vi "Analog Output Data Generation.vi"(3 "AO Timing":T1={"samples per channel"=1000, "sample mode"=10178, "Sampling Rate"=1000.0} {"sample mode" items=["Finite Samples"=10178, "Continuous Samples"=10123, "Hardware Timed Single Point"=12522]}, 4 "Configuration Data":T2[](array[typedef]), 5 "6738 Card?":bool, 6 "Path":path, 7 "AO Task":refnum<k21>, 8 "error in":errorcluster, 9 "Stop Notifier":refnum<notifier>, 10 "Main Engine Respons  Q":refnum<queue>, 11 "Interupt Q":refnum<queue>) -> (0 "error out":errorcluster, 2 "All Stop":bool)   [LabVIEW 2024]
doc: "All Rights Reserved © 2017 SyncSols"
uses:
  TCP Engine/Controls/TCP Engine I&O  Interupt Cluster.ctl
  Controls/AO Channel Configuration Cluster.ctl
  Controls/AO Timing Cluster.ctl
  <vilib>/DAQmx/write.llb/DAQmx Write (Analog 1D Wfm NChan NSamp).vi
  <vilib>/DAQmx/miscellaneous.llb/DAQmx Fill In Error Info.vi
  TCP Engine/TCP Engine.lvlib
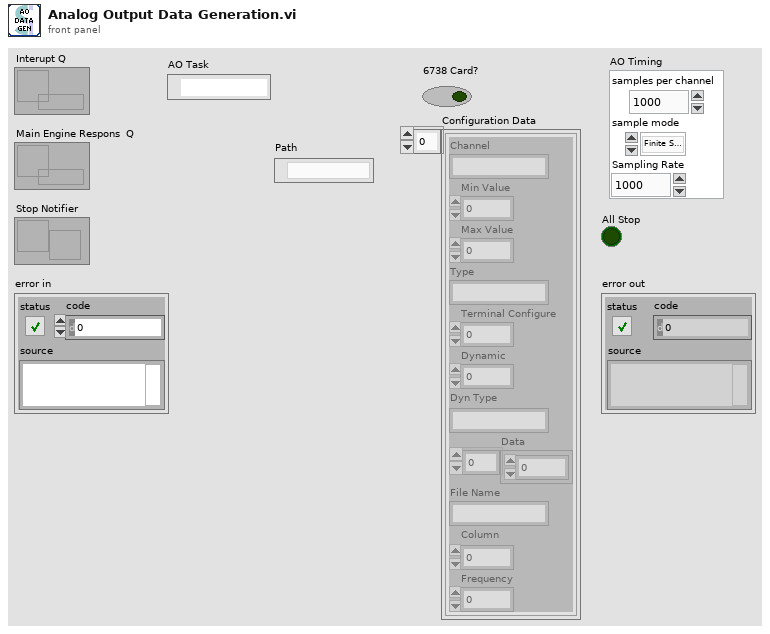
[diagram p1: front panel]
types:
  T1 = typedef "AO Timing Cluster.ctl" = cluster{"samples per channel":i32, "sample mode":i32, "Sampling Rate":dbl}
  T2 = typedef "AO Channel Configuration Cluster.ctl" = cluster{"Channel":string, "Min Value":dbl, "Max Value":dbl, "Type":string, "Terminal Configure":u16, "Dynamic":u8, "Dyn Type":string, "Data":dbl[], "File Name":string, "Column":i32, "Frequency":dbl}
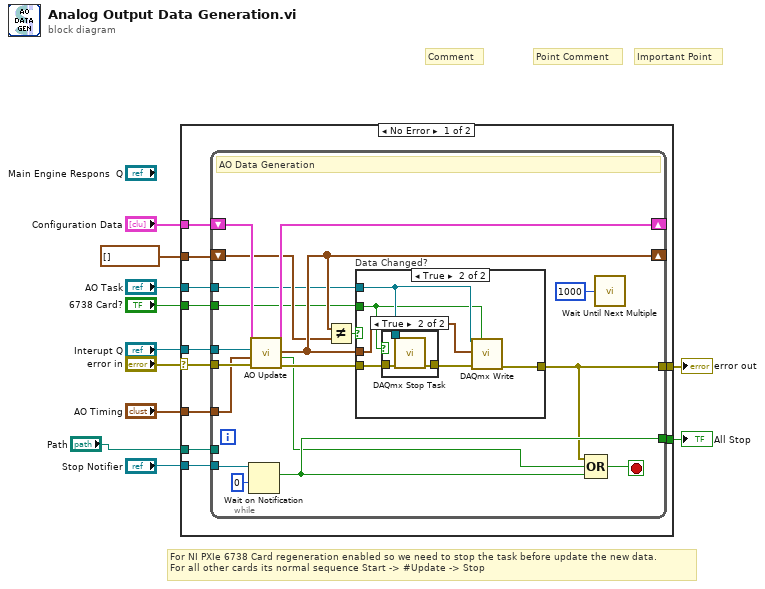
[diagram p0: block diagram]
diagram:
  # "For NI PXIe 6738 Card regeneration enabled so we need to stop the task before update the new data.\nFor all other cards its normal sequence Start -> #Update -> Stop"
  # "Important Point"
  # "Point Comment"
  # "Comment"
  n1 = case shown="No Error" "error in" {
    selector: "error in" -> [w20 w52]
    tunnel: [w18 w52] -> w11
    tunnel: "Stop Notifier" -> [w22 _]
    tunnel: "Interupt Q" -> [w21 _]
    tunnel: "AO Task" -> [w19 _]
    tunnel: "Path" -> [w17 _]
    tunnel: [w16 _] -> w7
    tunnel: "Configuration Data" -> [w15 _]
    tunnel: "AO Timing" -> [w14 _]
    tunnel: waveform(dbl)[] [] ("Data To Generate") -> [w13 _]
    tunnel: "6738 Card?" -> [w12 _]
    frame No Error {
      n2 = while {
        tunnel: w22 -> [w40]
        tunnel: w21 -> [w33]
        tunnel: w20 -> [w35]
        tunnel: w19 -> [w24]
        tunnel: [w29] -> w18
        tunnel: w17 -> [_]
        tunnel: [w37] -> w16
        tunnel: w14 -> [w32]
        shift-right: [w30] -> _
        shift-left: w15 -> [w34]
        shift-right: [w27] -> _
        shift-left: w13 -> [w26]
        tunnel: w12 -> [w23]
        stop <- w38 stop-if-true
        # "AO Data Generation"
        n3 = Wait on Notification(notifier=w40, timeout in ms (-1)=0) -> (notification=w37:bool)  [unwired: 2 in, 3 out]
        n4 = call "AO Update.vi"("error in"=w35, "AO Timing"=w32, "Interupt Q"=w33, "Configuration Data"=w34) -> ("error out"=w36:errorcluster, "Stop"=w31:bool, "Data To Generate"=w27:waveform(dbl)[], "Configuration Data"=w30:T2[])  [unwired: 4 in]
        n5 = Not Equal?(x=w27, y=w26) -> (x != y?=w28:bool)
        n6 = case "Data Changed?" shown="True" w28 {
          tunnel: w24 -> [_ w44]
          tunnel: w36 -> [w41 w45]
          tunnel: [w41 w47] -> w29
          tunnel: w27 -> [_ w46]
          tunnel: w23 -> [_ w42]
          frame False {
          }
          frame True {
            n7 = case shown="True" w42 {
              tunnel: w45 -> [w48 w51]
              tunnel: w44 -> [_ w50]
              tunnel: [w48 w49] -> w43
              frame False {
              }
              frame True {
                n8 = call <vilib>:"DAQmx Stop Task.vi"("task/channels in"=w50, "error in"=w51) -> ("error out"=w49:errorcluster)  [unwired: 12 in, 1 out]
              }
            }
            n9 = call-poly <vilib>:"DAQmx Write.vi"("task/channels in"=w44, "auto start"=w42, "data"=w46, "error in"=w43) -> ("error out"=w47:errorcluster)  [unwired: 9 in, 2 out]
          }
        }
        n10 = Compound Arithmetic op=OR(w29, w31, w37) -> (w38:bool)
        n11 = call "Wait Until Next Multiple"("Count(mSec)"=u32 1000) -> ()  [unwired: 1 out]
      }
    }
    frame Error {
    }
  }
  "error out" <- w11
  "All Stop" <- w7
